vi "RS.vi"(2 "S":bool, 3 "R":bool) -> (0 "nQ":bool, 1 "Q":bool)   [LabVIEW 2017]
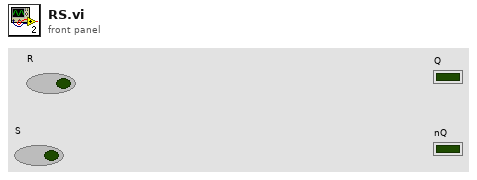
[diagram p1: front panel]
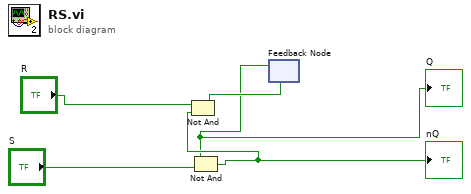
[diagram p0: block diagram]
diagram:
  n1 = feedback #1() -> (w1:bool)  [unwired: 1 in]
  "Q" <- w1
  n2 = Not And(1:"S", 2:w1) -> (0:w3:bool)
  "nQ" <- w3
  n3 = Not And(1:w3, 2:"R") -> (0:w2:bool)
  n4 = feedback-in #1(w2) -> ()
